vi "Init.vi"(4 "Name":string, 6 "Template Name":string, 8 "Template Path":path, 9 "Project:Active Project":refnum<vi>, 10 "NI.LV.Dialog Instance":refnum<vi>) -> (3 "Script out":refnum<class "_Template.lvclass">)   [LabVIEW 2021, in "_Template.lvlib" / "_Template.lvclass"]
uses:
  _Template.lvclass
  _Template.lvclass/_Template.ctl
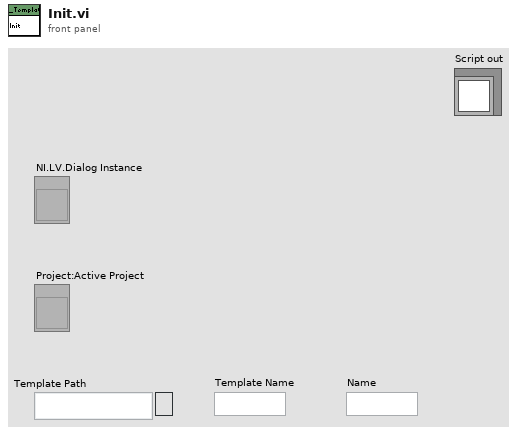
[diagram p1: front panel]
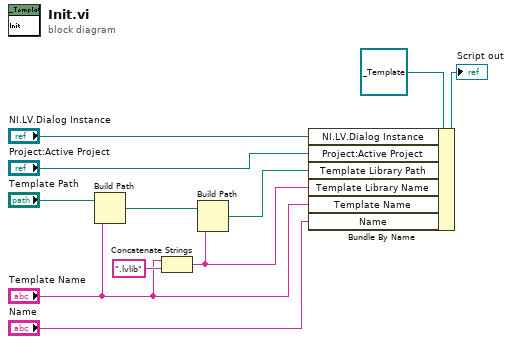
[diagram p0: block diagram]
diagram:
  n1 = Build Path(base path="Template Path", name or relative path="Template Name") -> (appended path=w9:path)
  n2 = Concatenate Strings("Template Name", ".lvlib" ("string")) -> (w1:string)
  n3 = Build Path(base path=w9, name or relative path=w1) -> (appended path=w7:path)
  n4 = Bundle By Name(cluster=refnum<class "_Template.lvclass"> refnum ("_Create From Template.lvlib:Script Strategy.lvlib:First Library Script Strategy.lvclass"), "NI.LV.Dialog Instance"="NI.LV.Dialog Instance", "Project:Active Project"="Project:Active Project", "Template Library Path"=w7, "Template Library Name"=w1, "Template Name"="Template Name", "Name"="Name") -> (→"Script out":refnum<class "_Template.lvclass">)
